vi "Write Parameters.vi"(8 "error in (no error)":errorcluster, 10 "Parameters":T1 {"Right Power" min=-1.0 max=1.0; "Left Power" min=-1.0 max=1.0}, 11 "Drive by Power in":refnum<class "Drive by Power.lvclass">) -> (0 "error out":errorcluster, 3 "Drive by Power out":refnum<class "Drive by Power.lvclass">)   [LabVIEW 2014, in "Forward Drive.lvlib" / "Drive by Power.lvclass"]
uses:
  Drive by Power.lvclass
  Parameters.ctl
  Drive by Power.lvclass/Drive by Power.ctl
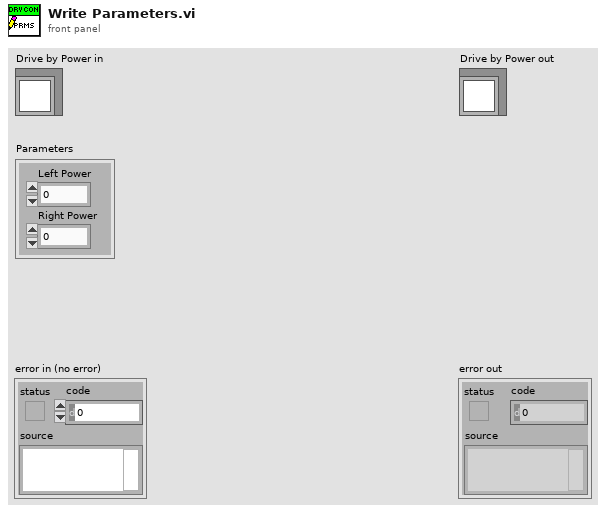
[diagram p1: front panel]
types:
  T1 = typedef "Forward Drive.lvlib/Drive by Power.lvclass/Parameters.ctl" = cluster{"Left Power":dbl, "Right Power ":dbl}
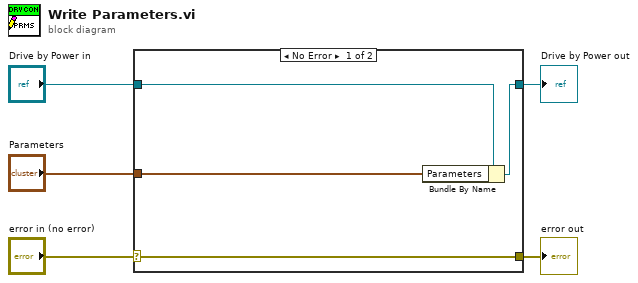
[diagram p0: block diagram]
diagram:
  n1 = case shown="No Error" "error in (no error)" {
    selector: "error in (no error)" -> [w9 w10]
    tunnel: [w9 w10] -> w4
    tunnel: [w7 w11] -> w2
    tunnel: "Drive by Power in" -> [w8 w11]
    tunnel: "Parameters" -> [w6 _]
    frame No Error {
      n2 = Bundle By Name(cluster=w8, "Parameters"=w6) -> (w7:refnum<class "Drive by Power.lvclass">)
    }
    frame Error {
    }
  }
  "error out" <- w4
  "Drive by Power out" <- w2
